vi "niDTS WLAN Dut Rx GetPacketsReceived.vi"(0 "Dut Handle in":T1, 11 "error in (no error)":errorcluster) -> (4 "Dut Handle out":T1, 6 "RX Packets Received":u32, 15 "error out":errorcluster)   [LabVIEW 2014, in "niDTS WLAN.lvlib"]
uses:
  niDTS WLAN.lvlib
  Framework/Dut/Includes/niDTS Dut INC Handle.ctl
  Framework/Dut/Objects/BASE_class/niDTS Dut.lvclass
  Includes/niDTS WLAN Dut INC Handle.ctl
  Objects/BASE_class/niDTS WLAN Dut.lvclass
  Framework/niDTS Framework.lvlib
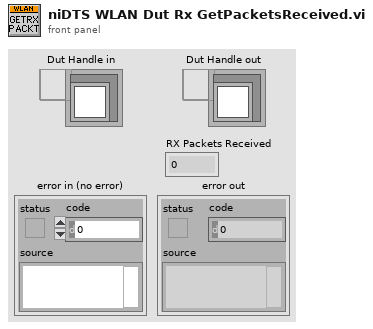
[diagram p1: front panel]
types:
  T1 = typedef "niDTS Framework.lvlib/niDTS Dut INC Handle.ctl" = refnum<data-value>
  T2 = typedef "niDTS WLAN.lvlib/niDTS WLAN Dut INC Handle.ctl" = refnum<data-value>
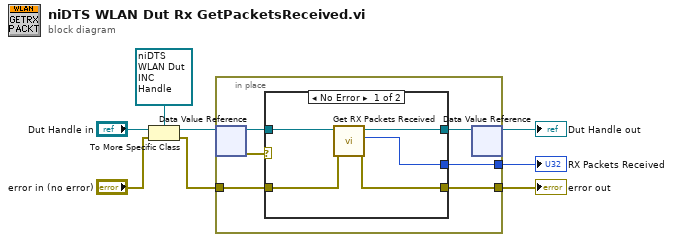
[diagram p0: block diagram]
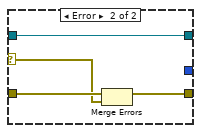
[diagram p2: hidden frame]
diagram:
  n1 = To More Specific Class(target class=T2 refnum ("WLAN Dut Handle"), reference="Dut Handle in", error in="error in (no error)") -> (specific class reference=w4:T2, error out=w2:errorcluster)
  n2 = in-place {
    in-place-border: w2 -> [w11]
    in-place-border: [w10] -> w7
    in-place-border: [w9] -> w1
    n3 = in-place-dvr #1(w4) -> (w13:refnum<class "niDTS WLAN Dut.lvclass">, w14:errorcluster)
    n4 = case shown="No Error" w14 {
      selector: w14 -> [_ w21]
      tunnel: w13 -> [w19 w23]
      tunnel: [w18 w23] -> w12
      tunnel: w11 -> [w16 w22]
      tunnel: [w17 w20] -> w10
      tunnel: [w15 _] -> w9
      frame No Error {
        n5 = call-dynamic "Get RX Packets Received.vi"("error in (no error)"=w16, "niDTS WLAN DUT in"=w19) -> ("error out"=w17:errorcluster, "RX Packets Received"=w15:u32, "niDTS WLAN DUT out"=w18:refnum<class "niDTS WLAN Dut.lvclass">)  [unwired: 7 in]
      }
      frame Error {
        n6 = Merge Errors(w22, w21) -> (w20:errorcluster)
      }
    }
    n7 = in-place-dvr #1(w12) -> (→"Dut Handle out":T2)  [unwired: 1 out]
  }
  "error out" <- w7
  "RX Packets Received" <- w1
